vi "Refresh Config Data from UDP.vi"(8 "error in (no error)":errorcluster, 10 "Timeout (2s)":dbl=2.0, 11 "Ethernet in":refnum<class "ENET_BS1201.lvclass">) -> (0 "error out":errorcluster, 1 "Received":bool, 2 "Configuration Data":string, 3 "Ethernet out":refnum<class "ENET_BS1201.lvclass">)   [LabVIEW 2021, in "BS120x Driver.lvlib" / "ENET_BS1201.lvclass"]
uses:
  ENET_BS1201.lvclass
  ENET_BS1201.lvclass/ENET_BS1201.ctl
panel:
  out "clear qty":i32
  out "Array":string[](array[string])
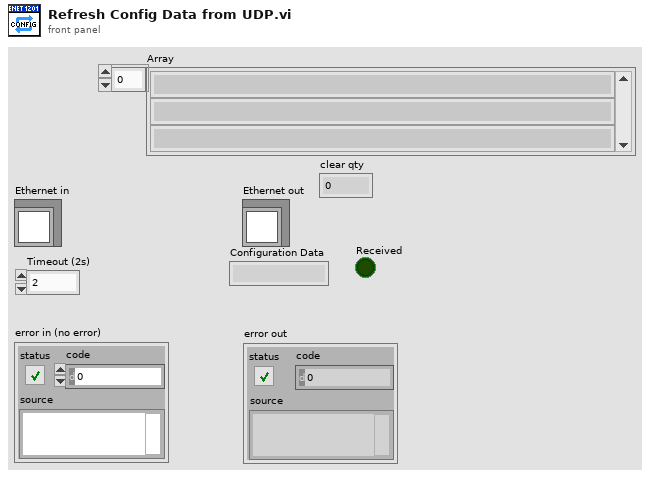
[diagram p1: front panel]
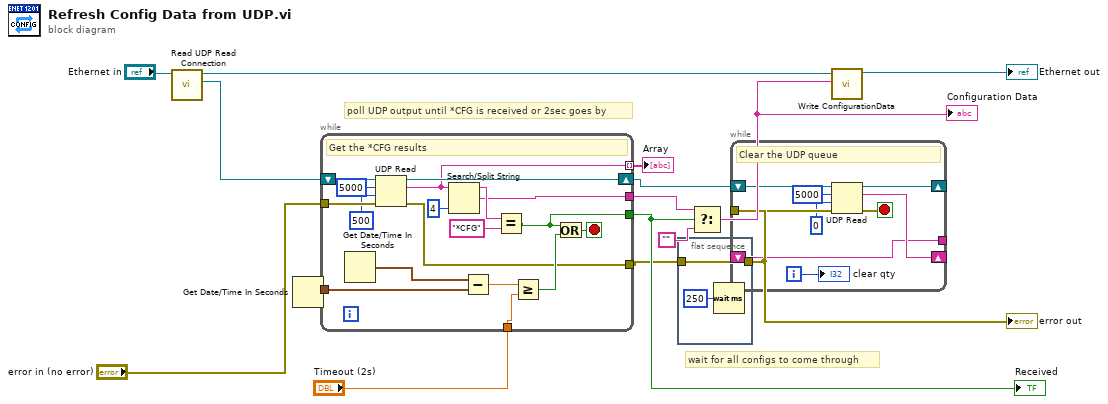
[diagram p0: block diagram]
diagram:
  # "wait for all configs to come through"
  # "poll UDP output until *CFG is received or 2sec goes by"
  n1 = call-dynamic "Read UDP Read Connection.vi"("ENET_BS120x in"="Ethernet in") -> ("UDP Read Connection"=w7:refnum<k16>, "ENET_BS120x out"=w6:refnum<class "ENET_BS1201.lvclass">)  [unwired: 8 in, 1 out]
  n2 = Get Date/Time In Seconds() -> (seconds since 1Jan1904=w14:timestamp)
  n3 = while {
    shift-right: [w31] -> w3
    shift-left: w7 -> [w32]
    tunnel: "error in (no error)" -> [w33]
    tunnel: [w18] -> w12
    tunnel: w14 -> [w27]
    tunnel: [w19] -> w13
    tunnel: [w23] -> w1
    tunnel: "Timeout (2s)" -> [w22]
    tunnel: [w17] -> w9 mode=indexing
    stop <- w25 stop-if-true
    # "Get the *CFG results"
    n4 = Get Date/Time In Seconds() -> (seconds since 1Jan1904=w28:timestamp)
    n5 = UDP Read(connection ID=w32, max size (548)=5000, timeout ms (25000)=500, 8:w33) -> (data out=w17:string, error out=w23:errorcluster, 3:w31:refnum<k16>)  [unwired: 2 out]
    n6 = Search/Split String(string=w17, offset (0)=4) -> (substring before match=w21:string, match + rest of string=w18:string)  [unwired: 1 in, 1 out]
    n7 = Subtract(x=w28, y=w27) -> (x-y=w26:dbl)
    n8 = Equal?(x=w21, y="*CFG") -> (x = y?=w19:bool)
    n9 = Greater Or Equal?(x=w26, y=w22) -> (x >= y?=w24:bool)
    n10 = Or(x=w19, y=w24) -> (x .or. y?=w25:bool)
  }
  "Received" <- w13
  "Array" <- w9
  n11 = flat-sequence {
    tunnel: [w35] -> w2
    tunnel: w1 -> [w35]
    frame #0 {
      n12 = Wait (ms)(milliseconds to wait=u32 250) -> ()  [unwired: 1 out]
    }
  }
  n13 = Select(t=w12, s=w13, f="") -> (s? t:f=w4:string)
  "Configuration Data" <- w4
  n14 = while {
    shift-right: [w42] -> _
    shift-left: w3 -> [w43]
    shift-right: [w41] -> _
    shift-left: _ -> [w38]
    tunnel: [w38] -> _
    tunnel: w2 -> [w44]
    i -> [w36]
    stop <- w39 stop-if-true
    # "Clear the UDP queue"
    n15 = UDP Read(connection ID=w43, max size (548)=5000, timeout ms (25000)=0, 8:w44) -> (data out=w41:string, error out=w39:errorcluster, 3:w42:refnum<k16>)  [unwired: 2 out]
    "clear qty" <- w36
  }
  n16 = call-dynamic "Write ConfigurationData.vi"("ConfigurationData"=w4, "ENET_BS120x in"=w6) -> ("ENET_BS120x out"=→"Ethernet out":refnum<class "ENET_BS1201.lvclass">)  [unwired: 8 in, 1 out]
  "error out" <- w2
